vi "Target Voltage Reached.vi"(8 "Error In":errorcluster, 9 "Time Target (s)":dbl=100.0, 10 "GEA Inputs":T1={"Source"=228, "Destination"=36} {"Destination" format="%.0x"; "Source" format="%.0x"}, 11 "GEA2 Reference In":refnum<k24>) -> (0 "error out":errorcluster, 1 "Report Text":string, 2 "Pass/Fail?":bool, 3 "GEA2 Reference Out":refnum<k24>)   [LabVIEW 2016]
uses:
  Q:/Common/DLLs/GEA3/GeaCommunication.dll
  Common/DLLs/GEA3/GeaCommunication.dll
  Common/LabVIEW GEA2 Toolkit/LabVIEW_GEA2_Toolkit.lvlibp/type defs/Source_Destination.ctl
  Common/LabVIEW GEA2 Toolkit/LabVIEW_GEA2_Toolkit.lvlibp/type defs/ERD Read Data In.ctl
  Common/LabVIEW GEA2 Toolkit/LabVIEW_GEA2_Toolkit.lvlibp/type defs/Data Type.ctl
  Common/LabVIEW GEA2 Toolkit/LabVIEW_GEA2_Toolkit.lvlibp
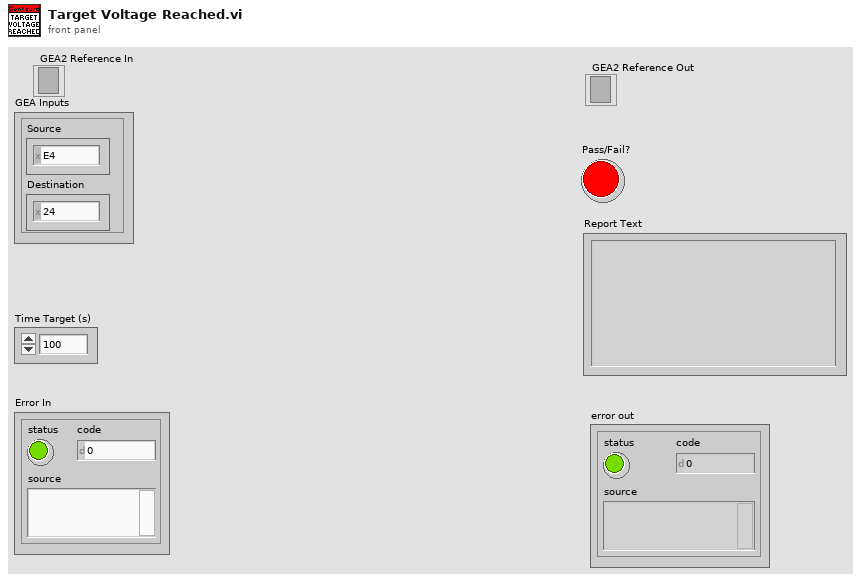
[diagram p1: front panel]
types:
  T1 = typedef "LabVIEW_GEA2_Toolkit.lvlibp/Source_Destination.ctl" = cluster{"Source":u8, "Destination":u8}
  T2 = typedef "LabVIEW_GEA2_Toolkit.lvlibp/ERD Read Data In.ctl" = cluster{"ERD Number":u16, "Data Type":T3}
  T3 = typedef "LabVIEW_GEA2_Toolkit.lvlibp/Data Type.ctl" = enum16{"string", "boolean", "uint8_t", "uint16_t", "uint32_t", "uint64_t", "int8_t", "int16_t", "int32_t", "int64_t"}
  T4 = typedef "LabVIEW_GEA2_Toolkit.lvlibp/ERD Read Data Out.ctl" = cluster{"ERD Number":u16, "Data":string}
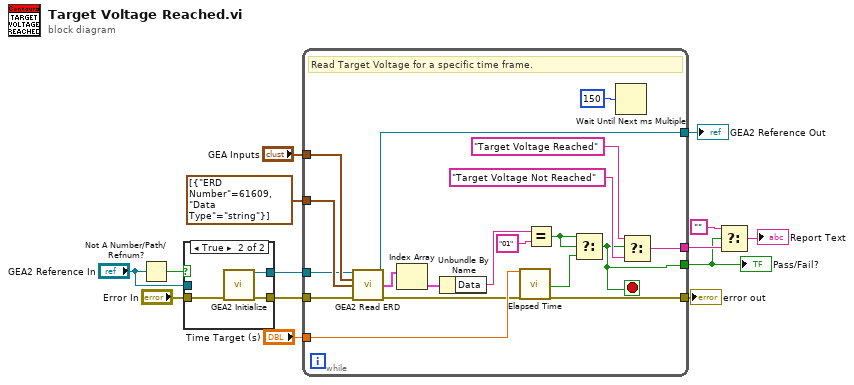
[diagram p0: block diagram]
diagram:
  n1 = Not A Number/Path/Refnum?(number/path/refnum="GEA2 Reference In") -> (NaN/Path/Refnum?=w12:bool)
  n2 = case shown="True" w12 {
    tunnel: [w15 w19] -> w9
    tunnel: "Error In" -> [w15 w18]
    tunnel: [w16 w17] -> w5
    tunnel: "GEA2 Reference In" -> [w16 _]
    frame False {
    }
    frame True {
      n3 = call "GEA2 Initialize.vi"("error in"=w18) -> ("GEA2 Reference Out"=w17:refnum<k24>, "error out"=w19:errorcluster)  [unwired: 12 in, 1 out]
    }
  }
  n4 = while {
    tunnel: w9 -> [w38]
    tunnel: T2[] [{"ERD Number"=61609, "Data Type"=enum."string"}] ("Read ERD List") -> [w37]
    tunnel: "GEA Inputs" -> [w36]
    tunnel: [w22] -> w6
    tunnel: w5 -> [w30]
    tunnel: "Time Target (s)" -> [w29]
    tunnel: [w26] -> w3
    tunnel: [w21] -> w2
    tunnel: [w20] -> w1
    stop <- w21 stop-if-true
    # "Read Target Voltage for a specific time frame."
    n5 = call "GEA2 Read ERD.vi"("GEA2 Reference In"=w30, "GEA Inputs"=w36, "Read ERD List"=w37, "Error In"=w38) -> ("GEA2 Reference Out"=w20:refnum<k24>, "ERD Data Out"=w35:T4[], "Error Out"=w23:errorcluster)  [unwired: 8 in, 1 out]
    n6 = Index Array(array=w35) -> (element=w34:T4)  [unwired: 1 in]
    n7 = Unbundle By Name(w34) -> ("Data"=w33:string)
    n8 = call "Elapsed Time"("Time Target (s)"=w29, "error in (no error)"=w23) -> ("Time has Elapsed"=w25:bool, "error out"=w22:errorcluster)  [unwired: 10 in, 6 out]
    n9 = Equal?(x=w33, y="01") -> (x = y?=w24:bool)
    n10 = Select(t=w24, s=w24, f=w25) -> (s? t:f=w21:bool)
    n11 = Wait Until Next ms Multiple(millisecond multiple=u32 150) -> ()  [unwired: 1 out]
    n12 = Select(t="Target Voltage Reached", s=w21, f="Target Voltage Not Reached") -> (s? t:f=w26:string)
  }
  "Pass/Fail?" <- w2
  "error out" <- w6
  "GEA2 Reference Out" <- w1
  n13 = Select(t="", s=w2, f=w3) -> (s? t:f=→"Report Text":string)
